vi "MotionProfileWriter.vi"(0 "PhoenixMotorControlDevRef":T6={"DeviceStatus"={"status"=FALSE, "code"=0, "source"=""}, "Type"=enum."PWM", "PWM"={"PWM Channel"=enum."Invalid", "DeadBand"={"Name"="", "maxPositivePwm"=0, "minPositivePwm"=0, "centerPwm"=0, "maxNegativePwm"=0, "minNegativePwm"=0, "angularRange"=0}}, "CAN"={"Device Number"=0, "SetOutput VI Ref"=variant(enum8{"Percent VBus", "Current", "Speed", "Position", "Voltage"} enum."Percent VBus"), "GetOutput VI Ref"=variant(refnum<k1> refnum), "Enable VI Ref"=variant(dbl 12.0), "Disable VI Ref"=variant(enum8{"Percent VBus", "Speed", "Position", "Slave", "Unchanged / Invalid", "Voltage Compensation", "Current", "Motion Profile"} enum."Percent VBus"), "Data"=variant}, "Invert"=FALSE, "DIO PWM"={"PWM \"Enable\" Channel"=enum."Invalid", "DIOChannel"=enum."Invalid", "PWM Rate"=0.0}}, 1 "ClearExistingMotionProfile":bool, 5 "Trajectory Points":T10[](array[typedef]) {"Time (ms)" items=["TrajectoryDuration_0ms"=0, "TrajectoryDuration_5ms"=5, "TrajectoryDuration_10ms"=10, "TrajectoryDuration_20ms"=20, "TrajectoryDuration_30ms"=30, "TrajectoryDuration_40ms"=40, "TrajectoryDuration_50ms"=50, "TrajectoryDuration_100ms"=100]}, 7 "MotorConfig":T1={"CAN Address"=0, "Invert"=FALSE, "InvertSensor"=FALSE, "Unit Conversion Factor"=0.0, "Brake Mode"=enum."Override to Brake", "Reverse Limt Switch Mode"=enum."Disabled", "Forward Limt Swith Mode"=enum."Disabled", "PWM Channel"=enum."Invalid", "Motor Controller Type"=enum."Talon SRX", "Peak Current (A)"=0, "Continuous Current (A)"=0, "Peak Duration (ms)"=0, "Current Limit Enable"=FALSE}, 9 "ProfileSlot0":i32, 11 "profileSlot1":i32, 12 "startIndex":i32) -> (4 "PhoenixMotorControlDevRef Out":T6={"DeviceStatus"={"status"=FALSE, "code"=0, "source"=""}, "Type"=enum."PWM", "PWM"={"PWM Channel"=enum."Invalid", "DeadBand"={"Name"="", "maxPositivePwm"=0, "minPositivePwm"=0, "centerPwm"=0, "maxNegativePwm"=0, "minNegativePwm"=0, "angularRange"=0}}, "CAN"={"Device Number"=0, "SetOutput VI Ref"=variant(enum8{"Percent VBus", "Current", "Speed", "Position", "Voltage"} enum."Percent VBus"), "GetOutput VI Ref"=variant(refnum<k1> refnum), "Enable VI Ref"=variant(dbl 12.0), "Disable VI Ref"=variant(enum8{"Percent VBus", "Speed", "Position", "Slave", "Unchanged / Invalid", "Voltage Compensation", "Current", "Motion Profile"} enum."Percent VBus"), "Data"=variant}, "Invert"=FALSE, "DIO PWM"={"PWM \"Enable\" Channel"=enum."Invalid", "DIOChannel"=enum."Invalid", "PWM Rate"=0.0}}, 15 "endIndex":i32)   [LabVIEW 2018, in "ArgosLib.lvlib"]
uses:
  ArgosLib.lvlib
  TypeDefs/TrajectoryPoint.ctl
  <vilib>/Rock Robotics/WPI/ThirdParty/Phoenix-LabVIEW/Motor Controller/Controls/CTRE_Phoenix_MotorControl_TrajectoryPointTimeDur.ctl
  <vilib>/Rock Robotics/WPI/MotorControl/WPI_MotorControlDeviceRef.ctl
  <vilib>/Rock Robotics/WPI/MotorControl/WPI_MotorControlType.ctl
  <vilib>/Rock Robotics/SystemInterfaces/DIO/FPGA_DIOPWMChannel.ctl
  <vilib>/Rock Robotics/WPI/PWM/WPI_PWMDeadband.ctl
  <vilib>/Rock Robotics/SystemInterfaces/DIO/FPGA_DIOChannel.ctl
  Config/ConfigComponents/TypeDefs/Config_Motor.ctl
  <vilib>/Rock Robotics/WPI/ThirdParty/Phoenix-LabVIEW/Motor Controller/Controls/CTRE_Phoenix_MotorControl_NeutralMode.ctl
  <vilib>/Rock Robotics/WPI/ThirdParty/Phoenix-LabVIEW/Motor Controller/Controls/CTRE_Phoenix_MotorControl_LimitSwitchNormal.ctl
  Config/ConfigComponents/TypeDefs/Config_MotorCtrlType.ctl
  <vilib>/Playing With Fusion Inc/Playing With Fusion Lib for FRC/PWF_Venom_LabVIEW/Public/TypeDefs/PwF_Venom_MPPoint.ctl
  <vilib>/Playing With Fusion Inc/Playing With Fusion Lib for FRC/PWF_Venom_LabVIEW/PwF_Venom.lvlib
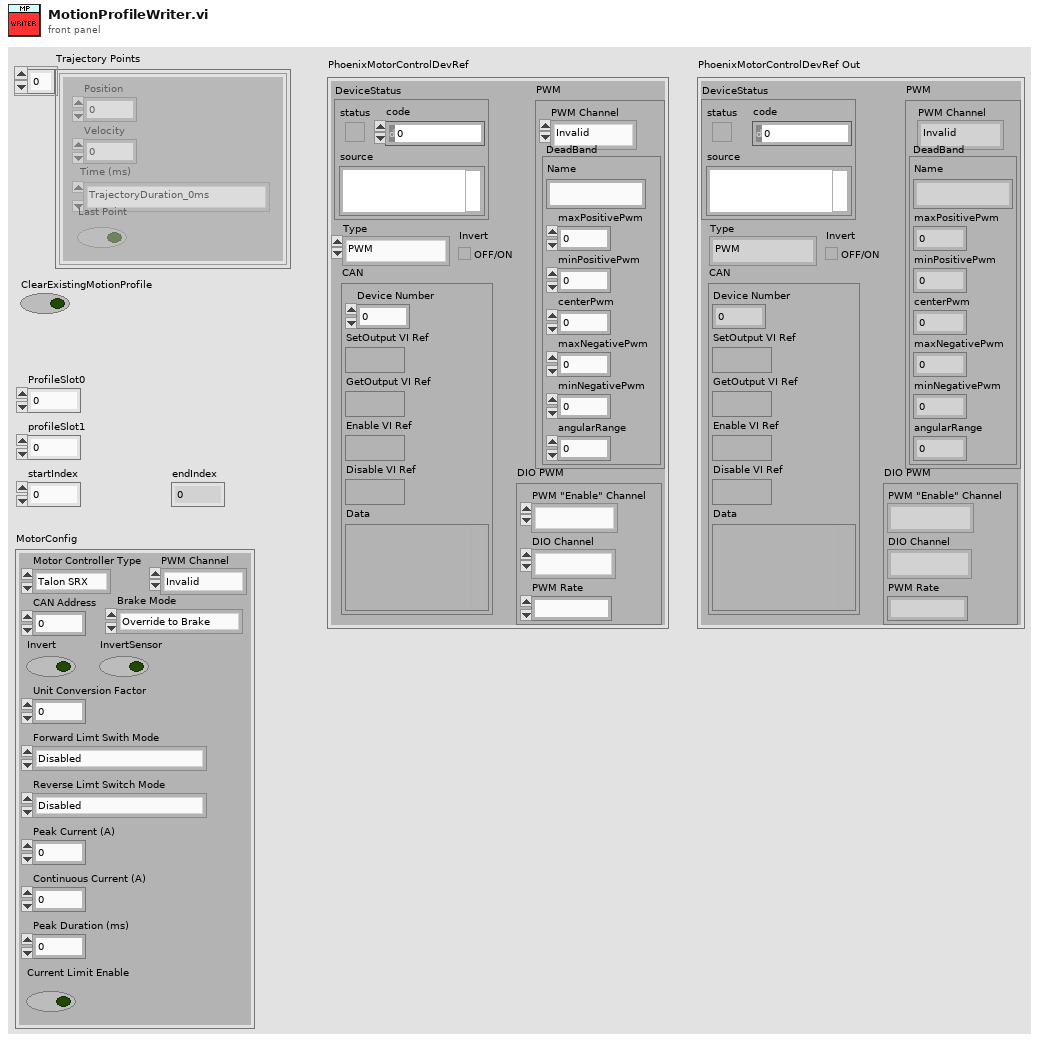
[diagram p1: front panel]
types:
  T1 = typedef "ArgosLib.lvlib/Config_Motor.ctl" = cluster{"CAN Address":u8, "Invert":bool, "InvertSensor":bool, "Unit Conversion Factor":dbl, "Brake Mode":T2, "Reverse Limt Switch Mode":T3, "Forward Limt Swith Mode":T3, "PWM Channel":T4, "Motor Controller Type":T5, "Peak Current (A)":i32, "Continuous Current (A)":i32, "Peak Duration (ms)":i32, "Current Limit Enable":bool}
  T2 = typedef "CTRE_Phoenix_MotorControl_NeutralMode.ctl" = enum8{"EEPROMSetting", "Override to Coast", "Override to Brake"}
  T3 = typedef "CTRE_Phoenix_MotorControl_LimitSwitchNormal.ctl" = enum16{"Normally Open", "Normally Closed", "Disabled"}
  T4 = typedef "FPGA_DIOPWMChannel.ctl" = enum8{"PWM 0", "PWM 1", "PWM 2", "PWM 3", "PWM 4", "PWM 5", "PWM 6", "PWM 7", "PWM 8", "PWM 9", "PWM MXP 0", "PWM MXP 1", "PWM MXP 2", "PWM MXP 3", "PWM MXP 4", "PWM MXP 5", "PWM MXP 6", "PWM MXP 7", "PWM MXP 8", "PWM MXP 9", "Invalid"}
  T5 = typedef "ArgosLib.lvlib/Config_MotorCtrlType.ctl" = enum16{"Disabled", "Talon SRX", "Talon SR", "Venom"}
  T6 = typedef "WPI_MotorControlDeviceRef.ctl" = cluster{"DeviceStatus":errorcluster, "Type":T7, "PWM":cluster{"PWM Channel":T4, "DeadBand":T8}, "CAN":cluster{"Device Number":u8, "SetOutput VI Ref":variant, "GetOutput VI Ref":variant, "Enable VI Ref":variant, "Disable VI Ref":variant, "Data":variant}, "Invert":bool, "DIO PWM":cluster{"PWM \"Enable\" Channel":T4, "DIOChannel":T9, "PWM Rate":dbl}}
  T7 = typedef "WPI_MotorControlType.ctl" = enum16{"PWM", "CAN", "DIO PWM"}
  T8 = typedef "WPI_PWMDeadband.ctl" = cluster{"Name":string, "maxPositivePwm":i32, "minPositivePwm":i32, "centerPwm":i32, "maxNegativePwm":i32, "minNegativePwm":i32, "angularRange":u16}
  T9 = typedef "FPGA_DIOChannel.ctl" = enum8{"DIO 0", "DIO 1", "DIO 2", "DIO 3", "DIO 4", "DIO 5", "DIO 6", "DIO 7", "DIO 8", "DIO 9", "DIO MXP 0", "DIO MXP 1", "DIO MXP 2", "DIO MXP 3", "DIO MXP 4", "DIO MXP 5", "DIO MXP 6", "DIO MXP 7", "DIO MXP 8", "DIO MXP 9", "DIO MXP 10", "DIO MXP 11", "DIO MXP 12", "DIO MXP 13", "DIO MXP 14", "DIO MXP 15", "SPI Port CS1", "SPI Port CS2", "SPI Port CS3", "SPI Port MISO", "SPI Port MOSI", "Invalid"}
  T10 = typedef "ArgosLib.lvlib/TrajectoryPoint.ctl" = cluster{"Position ":dbl, "Velocity ":dbl, "Time (ms)":T11, "Last Point":bool}
  T11 = typedef "CTRE_Phoenix_MotorControl_TrajectoryPointTimeDur.ctl" = i32
  T12 = cluster{"Top Buffer Remaining":i32, "Top Buffer Count":i32, "Bottom Buffer Count":i32, "Has Underrun?":bool, "Is Underrun?":bool, "Active Point Valid?":bool, "Is Last?":bool, "Profile Slot Select 0":i32, "Output Enable":i32, "Time Duration (ms)":i32, "Profile Slot Select 1":i32}
  T13 = typedef "PlayingWithFusionLib.lvlib/PwF_Venom.lvlib/PwF_Venom_MPPoint.ctl" = cluster{"Time":dbl, "Speed":dbl, "Position":dbl}
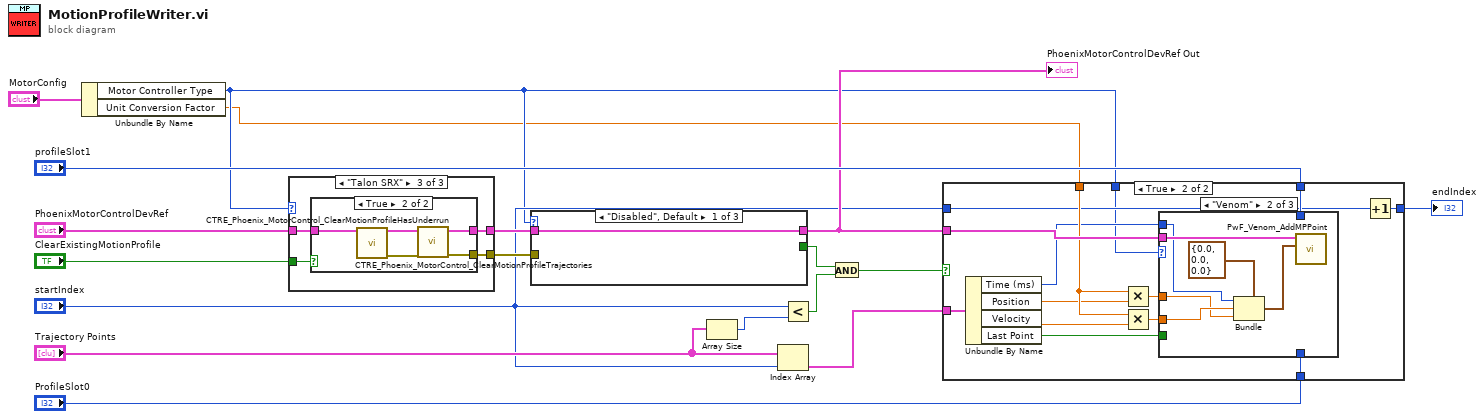
[diagram p0: block diagram]
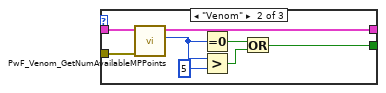
[diagram p2: hidden frame]
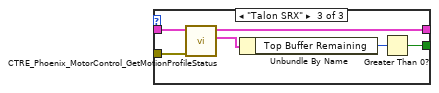
[diagram p3: hidden frame]
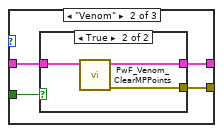
[diagram p5: hidden frame]
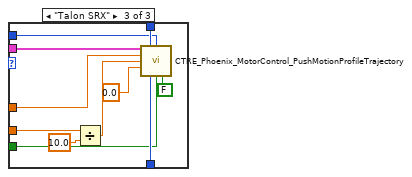
[diagram p10: hidden frame]
diagram:
  n1 = Unbundle By Name("MotorConfig") -> ("Motor Controller Type"=w2:T5, "Unit Conversion Factor"=w1:dbl)
  n2 = case shown="\"Talon SRX\"" w2 {
    tunnel: "ClearExistingMotionProfile" -> [_ w20 w31]
    tunnel: "PhoenixMotorControlDevRef" -> [w19 w23 w30]
    tunnel: [w19 w22 w29] -> w14
    tunnel: [_ w21 w28] -> w13
    frame "Disabled", Default {
    }
    frame "Venom" {
      n3 = case shown="True" w20 {
        tunnel: w23 -> [w24 w27]
        tunnel: [w24 w26] -> w22
        tunnel: [_ w25] -> w21
        frame False {
        }
        frame True {
          n4 = call <vilib>:"PwF_Venom_ClearMPPoints.vi"("PwFVenomDevRefIn"=w27) -> ("error out"=w25:errorcluster, "PwFVenomDevRefOut"=w26:T6)  [unwired: 9 in]
        }
      }
    }
    frame "Talon SRX" {
      n5 = case shown="True" w31 {
        tunnel: w30 -> [w32 w37]
        tunnel: [w32 w33] -> w29
        tunnel: [_ w34] -> w28
        frame False {
        }
        frame True {
          n6 = call <vilib>:"CTRE_Phoenix_MotorControl_ClearMotionProfileTrajectories.vi"("PhoenixMotorControlDevRef"=w37) -> ("PhoenixMotorControlDevRef"=w36:T6, "error out"=w35:errorcluster)  [unwired: 13 in]
          n7 = call <vilib>:"CTRE_Phoenix_MotorControl_ClearMotionProfileHasUnderrun.vi"("error in"=w35, "PhoenixMotorControlDevRef"=w36) -> ("error out"=w34:errorcluster, "PhoenixMotorControlDevRef"=w33:T6)  [unwired: 8 in]
        }
      }
    }
  }
  n8 = case shown="\"Disabled\", Default" w2 {
    tunnel: w14 -> [w38 w45 w52]
    tunnel: w13 -> [_ w46 w50]
    tunnel: [w38 w44 w49] -> w12
    tunnel: [_ w39 w47] -> w5
    frame "Disabled", Default {
    }
    frame "Venom" {
      n9 = call <vilib>:"PwF_Venom_GetNumAvailableMPPoints.vi"("error in"=w46, "PwFVenomDevRefIn"=w45) -> ("Available MP Points"=w41:u16, "PwFVenomDevRefOut"=w44:T6)  [unwired: 7 in, 1 out]
      n10 = Equal To 0?(x=w41) -> (x = 0?=w43:bool)
      n11 = Greater?(x=w41, y=u16 5) -> (0:w42:bool)
      n12 = Or(x=w43, y=w42) -> (x .or. y?=w39:bool)
    }
    frame "Talon SRX" {
      n13 = call <vilib>:"CTRE_Phoenix_MotorControl_GetMotionProfileStatus.vi"("error in"=w50, "PhoenixMotorControlDevRef"=w52) -> ("Motion Profile Status"=w51:T12, "PhoenixMotorControlDevRef"=w49:T6)  [unwired: 7 in, 1 out]
      n14 = Unbundle By Name(w51) -> ("Top Buffer Remaining"=w48:i32)
      n15 = Greater Than 0?(x=w48) -> (x > 0?=w47:bool)
    }
  }
  "PhoenixMotorControlDevRef Out" <- w12
  n16 = Array Size(array="Trajectory Points") -> (size(s)=w8:i32)
  n17 = Index Array(array="Trajectory Points", index="startIndex") -> (element=w11:T10)
  n18 = Less?(x="startIndex", y=w8) -> (x < y?=w6:bool)
  n19 = And(x=w5, y=w6) -> (x .and. y?=w4:bool)
  n20 = case shown="True" w4 {
    tunnel: "ProfileSlot0" -> [_ w67]
    tunnel: "profileSlot1" -> [_ w66]
    tunnel: w12 -> [_ w65]
    tunnel: w1 -> [_ w64]
    tunnel: w11 -> [_ w57]
    tunnel: "startIndex" -> [w53 w56]
    tunnel: [w53 w55] -> w10
    tunnel: w2 -> [_ w54]
    frame False {
    }
    frame True {
      n21 = Unbundle By Name(w57) -> ("Time (ms)"=w62:T11, "Position"=w60:dbl, "Velocity"=w59:dbl, "Last Point"=w63:bool)
      n22 = Multiply(x=w64, y=w60) -> (x*y=w61:dbl)
      n23 = Multiply(x=w64, y=w59) -> (x*y=w58:dbl)
      n24 = case shown="\"Venom\"" w54 {
        tunnel: w67 -> [_ _ w84]
        tunnel: w66 -> [_ _ w83]
        tunnel: w65 -> [_ w73 w82]
        tunnel: w63 -> [_ _ w81]
        tunnel: w62 -> [_ w69 w80]
        tunnel: w61 -> [_ w70 w77]
        tunnel: w58 -> [_ w71 w75]
        frame "Disabled", Default {
        }
        frame "Venom" {
          n25 = Bundle(cluster=T13 {"Time"=0.0, "Speed"=0.0, "Position"=0.0} ("Motion Profile Point"), "Time"=w69, "Speed"=w71, "Position"=w70) -> (w68:T13)
          n26 = call <vilib>:"PwF_Venom_AddMPPoint.vi"("Motion Profile Point"=w68, "PwFVenomDevRefIn"=w73) -> ()  [unwired: 8 in, 2 out]
        }
        frame "Talon SRX" {
          n27 = Divide(x=w75, y=10.0) -> (x/y=w74:dbl)
          n28 = call <vilib>:"CTRE_Phoenix_MotorControl_PushMotionProfileTrajectory.vi"("PhoenixMotorControlDevRef"=w82, "profileSlotSelect1"=w83, "durationMs"=w80, "position"=w77, "velocity"=w74, "auxiliaryPos"=0.0 ("headingDeg"), "profileSlotSelect0"=w84, "isLastPoint?"=w81, "Zero Position?"=FALSE) -> ()  [unwired: 5 in, 2 out]
        }
      }
      n29 = Increment(x=w56) -> (x+1=w55:i32)
    }
  }
  "endIndex" <- w10
